vi "IQ vs Slot Measurement Overall Frequency Error Error Codes.vi"(8 "error in (no error)":errorcluster, 9 "Instance (1)":i32=1, 11 "VISA resource name":refnum<visa-resource-name>) -> (0 "error out":errorcluster, 1 "Error Codes":i32[](array[numeric]), 2 "Reliability":i32, 3 "VISA resource name out":refnum<visa-resource-name>)   [LabVIEW 2015, in "Rohde&Schwarz CMXP GPRF.lvlib"]
doc: "Returns a single-value error code for each result.\n\nAttribute:\nRSCMXPGPRF_ATTR_IQ_VS_SLOT_MEASUREMENT_OVERALL_FREQUENCY_ERROR_LIMIT_CHECK_RESULT\n\nRemote-control command:\nCALCulate:GPRF:MEAS<i>:IQVSlot:OFERror?"
uses:
  <instrlib>/Rohde&Schwarz CMXP GPRF/Rohde&Schwarz CMXP GPRF.lvlib
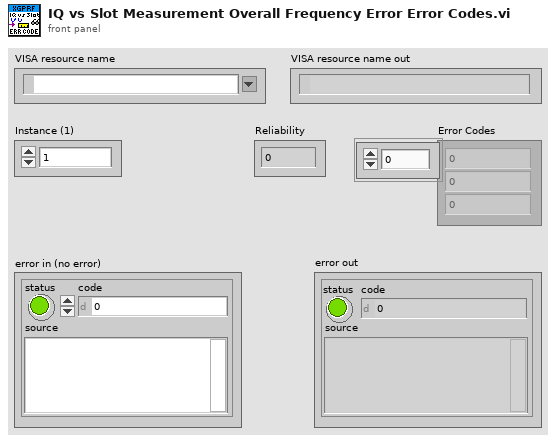
[diagram p1: front panel]
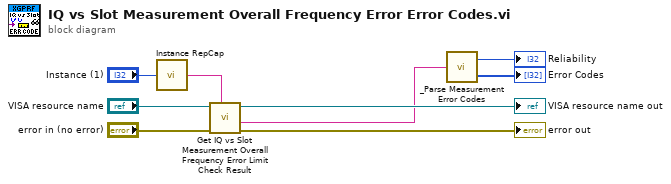
[diagram p0: block diagram]
diagram:
  n1 = call <instrlib>:"Instance RepCap.vi"("instance  in"="Instance (1)") -> ("instance out"=w4:string)
  n2 = call "Get IQ vs Slot Measurement Overall Frequency Error Limit Check Result"("Repeated Capabilities"=w4, "error in (no error)"="error in (no error)", "instrument handle"="VISA resource name") -> ("error out"=→"error out":errorcluster, "IQ vs Slot Measurement Overall Frequency Error Limit Check Result"=w1:string, "instrument handle out"=→"VISA resource name out":refnum<visa-resource-name>)  [unwired: 6 in]
  n3 = call <instrlib>:"_Parse Measurement Error Codes.vi"("String In"=w1) -> ("Reliability"=→"Reliability":i32, "Results"=→"Error Codes":i32[])
